vi "Test TCRS Cools Down While Disabled Before Restarting Heating.vi"(8 "error in (no error)":errorcluster, 11 "Thermal Chamber Response Simlator Test In":refnum<class "Thermal Chamber Response Simlator Test.lvclass">) -> (0 "error out":errorcluster, 3 "Thermal Chamber Response Simlator Test Out":refnum<class "Thermal Chamber Response Simlator Test.lvclass">)   [LabVIEW 2020, in "Thermal Chamber Response Simlator Test.lvclass"]
uses:
  Thermal Chamber Response Simlator Test.lvclass
  C:/Program Files (x86)/National Instruments/LabVIEW 2020/vi.lib/Asteme/LUnit/Test Case.lvclass
  Thermal Chamber Response Simlator/Thermal Chamber Response Simlator.lvclass
  Thermal Chamber Response Simlator/Thermal Chamber Response Simlator.lvclass/Thermal Chamber Response Simlator.ctl
  <vilib>/Asteme/LUnit/Test Case.lvclass/Test Case.ctl
  <vilib>/Asteme/LUnit/LUnit Assertion Result.lvclass/LUnit Assertion Result.ctl
  <vilib>/Asteme/LUnit/Palette/Fail.vi
  <vilib>/Asteme/LUnit/Palette/Pass.vi
  <vilib>/Asteme/LUnit/Set Assertion Type.vi
  <vilib>/Asteme/LUnit/Add test result.vi
  <vilib>/Asteme/LUnit/LUnit Write Passed.vi
  <vilib>/Asteme/LUnit/LUnit Get Test Case.vi
  <vilib>/Asteme/LUnit/Assertion Result/LUnit Get Test Name.vi
  <vilib>/Asteme/LUnit/LUnit Write Message.vi
  <vilib>/Asteme/LUnit/LUnit Write Description.vi
  <vilib>/Asteme/LUnit/LUnit Write Assertion Type.vi
  <vilib>/Asteme/LUnit/Read Test Case Name.vi
  Thermal Chamber Response Simlator/Private/Get Current Time if Not Set.vi
  <vilib>/Asteme/LUnit/LUnit Assertion Result.lvclass
  <vilib>/Asteme/LUnit/Test Case.lvclass
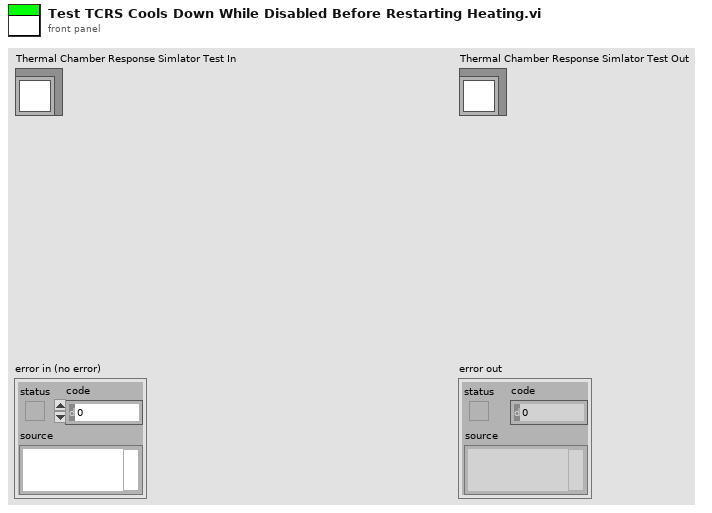
[diagram p1: front panel]
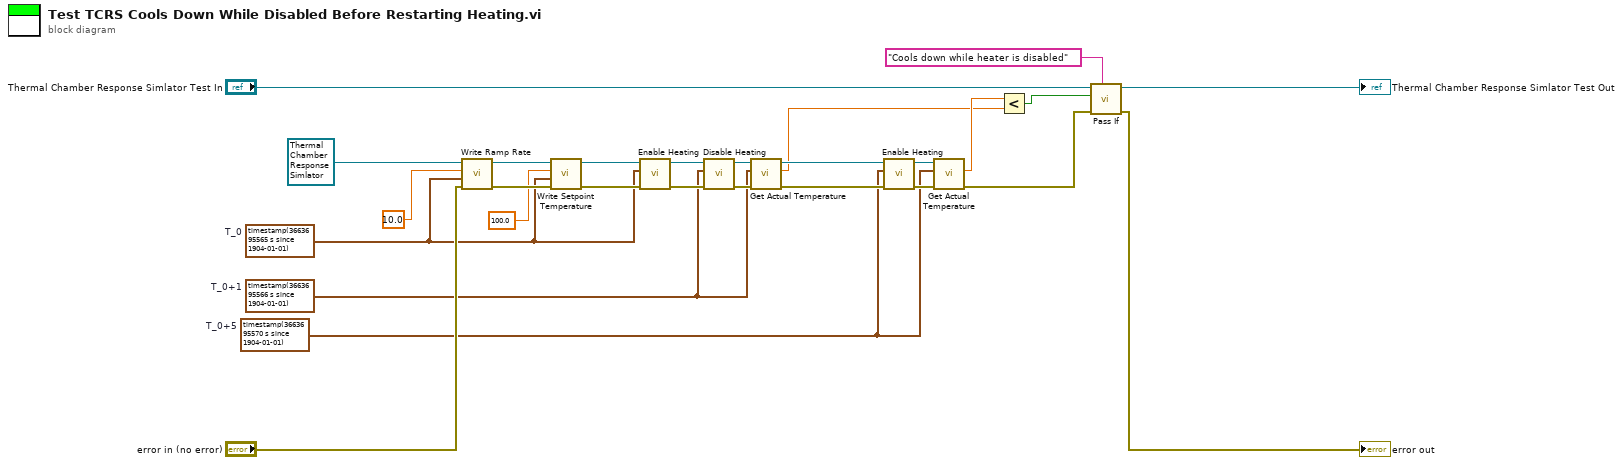
[diagram p0: block diagram]
diagram:
  w2 = timestamp(3663695570 s since 1904-01-01)  # T_0+5
  w16 = timestamp(3663695566 s since 1904-01-01)  # T_0+1
  w1 = timestamp(3663695565 s since 1904-01-01)  # T_0
  n1 = call "Write Ramp Rate.vi"("error in (no error)"="error in (no error)", "Time Stamp"=w1, "Ramp Rate [degC/s]"=10.0, "Thermal Chamber Response Simlator In"=refnum<class "Thermal Chamber Response Simlator.lvclass"> refnum ("Thermal Chamber Response Simlator.lvclass")) -> ("error out"=w26:errorcluster, "Thermal Chamber Response Simlator Out"=w13:refnum<class "Thermal Chamber Response Simlator.lvclass">)  [unwired: 6 in]
  n2 = call "Write Setpoint Temperature.vi"("error in (no error)"=w26, "Update Time"=w1, "Setpoint Temperature [degC]"=100.0, "Thermal Chamber Response Simlator In"=w13) -> ("error out"=w14:errorcluster, "Thermal Chamber Response Simlator Out"=w12:refnum<class "Thermal Chamber Response Simlator.lvclass">)  [unwired: 6 in]
  n3 = call "Enable Heating.vi"("error in (no error)"=w14, "Start Time"=w1, "Thermal Chamber Response Simlator In"=w12) -> ("error out"=w23:errorcluster, "Thermal Chamber Response Simlator Out"=w24:refnum<class "Thermal Chamber Response Simlator.lvclass">)  [unwired: 7 in]
  n4 = call "Disable Heating.vi"("error in (no error)"=w23, "Start Time"=w16, "Thermal Chamber Response Simlator In"=w24) -> ("error out"=w21:errorcluster, "Thermal Chamber Response Simlator Out"=w22:refnum<class "Thermal Chamber Response Simlator.lvclass">)  [unwired: 7 in]
  n5 = call "Get Actual Temperature.vi"("error in (no error)"=w21, "Time Stamp"=w16, "Thermal Chamber Response Simlator In"=w22) -> ("error out"=w20:errorcluster, "Actual Temperature [degC]"=w5:dbl, "Thermal Chamber Response Simlator Out"=w18:refnum<class "Thermal Chamber Response Simlator.lvclass">)  [unwired: 6 in]
  n6 = call "Enable Heating.vi"("error in (no error)"=w20, "Start Time"=w2, "Thermal Chamber Response Simlator In"=w18) -> ("error out"=w19:errorcluster, "Thermal Chamber Response Simlator Out"=w17:refnum<class "Thermal Chamber Response Simlator.lvclass">)  [unwired: 7 in]
  n7 = call "Get Actual Temperature.vi"("error in (no error)"=w19, "Time Stamp"=w2, "Thermal Chamber Response Simlator In"=w17) -> ("error out"=w10:errorcluster, "Actual Temperature [degC]"=w6:dbl)  [unwired: 6 in, 1 out]
  n8 = Less?(x=w6, y=w5) -> (x < y?=w4:bool)
  n9 = call <vilib>:"Pass If.vi"("Description"="Cools down while heater is disabled", "error in (no error)"=w10, "Pass?"=w4, "Test Case In"="Thermal Chamber Response Simlator Test In") -> ("error out"=→"error out":errorcluster, "Test Case Out"=→"Thermal Chamber Response Simlator Test Out":refnum<class "Thermal Chamber Response Simlator Test.lvclass">)  [unwired: 6 in]
